vi "Interpret Packet Header.vi"(11 "input data":bool[](array[boolean])) -> (1 "reserved_bits":bool[](array[boolean]), 2 "timestamp":u64, 3 "chdr_header":T1)   [LabVIEW 2023, in "CHDR Support.lvlib"]
doc: "Parses a 256-bit CHDR header into a readable cluster."
uses:
  CHDR Support.lvlib
  CHDR Header Layout.ctl
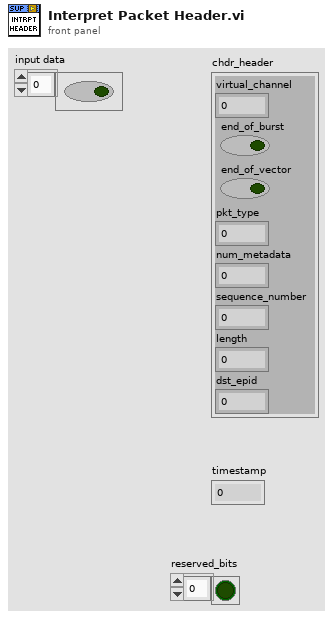
[diagram p1: front panel]
types:
  T1 = typedef "CHDR Support.lvlib/CHDR Header Layout.ctl" = cluster{"virtual_channel":fxp<+,6,6>, "end_of_burst":bool, "end_of_vector":bool, "pkt_type":fxp<+,3,3>, "num_metadata":fxp<+,5,5>, "sequence_number":u16, "length":u16, "dst_epid":u16}
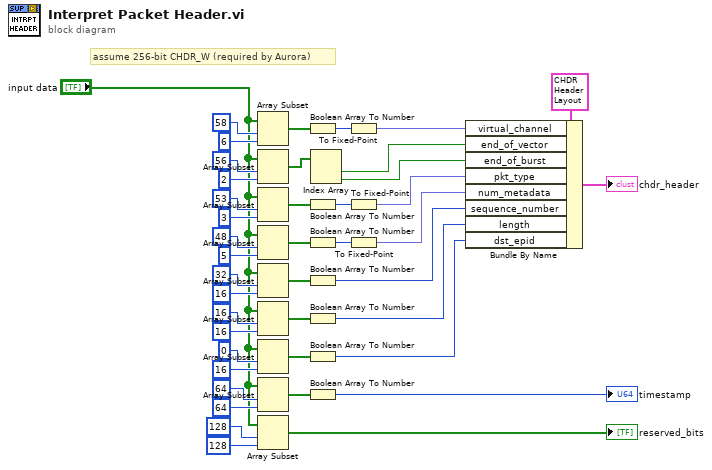
[diagram p0: block diagram]
diagram:
  # "assume 256-bit CHDR_W (required by Aurora)"
  n1 = Array Subset(array="input data", index=58, length=6) -> (w42:bool[])
  n2 = Array Subset(array="input data", index=56 ("length"), length=2) -> (w41:bool[])
  n3 = Array Subset(array="input data", index=53 ("length"), length=3) -> (w40:bool[])
  n4 = Array Subset(array="input data", index=48 ("length"), length=5) -> (w39:bool[])
  n5 = Array Subset(array="input data", index=32 ("length"), length=16) -> (w38:bool[])
  n6 = Array Subset(array="input data", index=16 ("length"), length=16) -> (w37:bool[])
  n7 = Array Subset(array="input data", index=0 ("length"), length=16) -> (w36:bool[])
  n8 = Array Subset(array="input data", index=64 ("length"), length=64) -> (w35:bool[])
  n9 = Array Subset(array="input data", index=128 ("length"), length=128) -> (→"reserved_bits":bool[])
  n10 = Boolean Array To Number(Boolean array=w42) -> (number=w29:u8)
  n11 = Boolean Array To Number(Boolean array=w40) -> (number=w28:u8)
  n12 = Boolean Array To Number(Boolean array=w39) -> (number=w27:u8)
  n13 = Boolean Array To Number(Boolean array=w38) -> (number=w21:u16)
  n14 = Boolean Array To Number(Boolean array=w37) -> (number=w20:u16)
  n15 = Boolean Array To Number(Boolean array=w36) -> (number=w23:u16)
  n16 = Boolean Array To Number(Boolean array=w35) -> (number=→"timestamp":u64)
  n17 = Index Array(array=w41) -> (element #1=w34:bool, element #2=w33:bool)  [unwired: 2 in]
  n18 = To Fixed-Point(number=w29) -> (fixed-point=w26:fxp<+,6,6>)  [unwired: 1 in]
  n19 = To Fixed-Point(number=w28) -> (fixed-point=w25:fxp<+,3,3>)  [unwired: 1 in]
  n20 = To Fixed-Point(number=w27) -> (fixed-point=w24:fxp<+,5,5>)  [unwired: 1 in]
  n21 = Bundle By Name(cluster=T1 {"virtual_channel"=0.0, "end_of_burst"=FALSE, "end_of_vector"=FALSE, "pkt_type"=0.0, "num_metadata"=0.0, "sequence_number"=0, "length"=0, "dst_epid"=0} ("chdr_header"), "virtual_channel"=w26, "end_of_vector"=w34, "end_of_burst"=w33, "pkt_type"=w25, "num_metadata"=w24, "sequence_number"=w21, "length"=w20, "dst_epid"=w23) -> (→"chdr_header":T1)
